vi "Call WFG Plug In.vi"(8 "Parameters":variant, 9 "Frequency":dbl, 10 "Amplitude":dbl, 11 "Plug-in VI Path":path) -> (3 "Signal out":waveform(dbl))   [LabVIEW 2011]
doc: "This VI calls the valid plug ins that are of the type that is specified by the strict type def control. It calls VIs that are used in the plug in exercise.\n\nAAL 9/09"
panel:
  in  "VI Refnum (type only)":refnum<vi>
  out "error out":errorcluster
  in  "error in (no error)":errorcluster
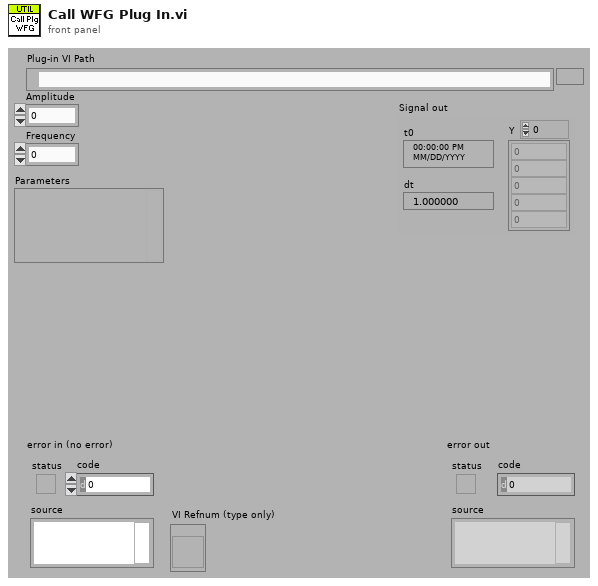
[diagram p1: front panel]
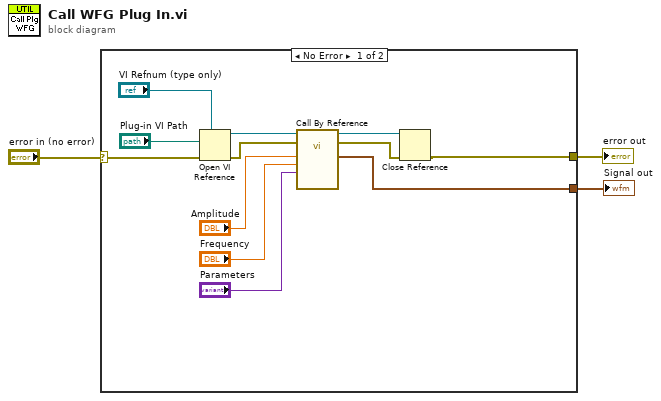
[diagram p0: block diagram]
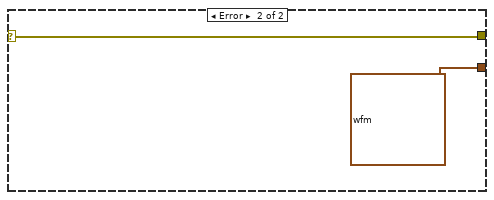
[diagram p2: hidden frame]
diagram:
  n1 = case shown="No Error" "error in (no error)" {
    selector: "error in (no error)" -> [w11 w17]
    tunnel: [w4 w17] -> w2
    tunnel: [w5 waveform(dbl) {"t0"=timestamp(0 s since 1904-01-01), "dt"=1.0, "Y"=[]} ("Signal out")] -> w1
    frame No Error {
      n2 = Open VI Reference(type specifier VI Refnum (for type only)="VI Refnum (type only)", vi path="Plug-in VI Path", error in (no error)=w11) -> (vi reference=w13:refnum<vi>, error out=w10:errorcluster)  [unwired: 3 out]
      n3 = call-by-ref "?"(reference=w13, error in=w10, "Parameters"="Parameters", "Frequency"="Frequency", "Amplitude"="Amplitude") -> (reference out=w12:refnum<vi>, error out=w9:errorcluster, "Signal out"=w5:waveform(dbl))  [unwired: 8 in]
      n4 = Close Reference(reference=w12, error in (no error)=w9) -> (error out=w4:errorcluster)
    }
    frame Error {
    }
  }
  "error out" <- w2
  "Signal out" <- w1
